vi "IB_RW_Project_RegGroup.vi"(7 "action":T3, 8 "error in (no error)":errorcluster, 9 "index in":string, 10 "RegGroup":T2, 11 "buildObject":T1) -> (0 "error out":errorcluster, 1 "index out":string, 2 "RegGroup":T2, 3 "buildObject out":T1)   [LabVIEW 2020]
doc: "Reads and writes the data to the object property bag."
uses:
  <resource>/Framework/Providers/API/ItemRef.ctl
  <vilib>/AppBuilder/IB_RW_Project/IB_RW_Project_PropBag_Action.ctl
  <vilib>/AppBuilder/IB_RW_Project/IB_RW_Project_RegGroup_Data.ctl
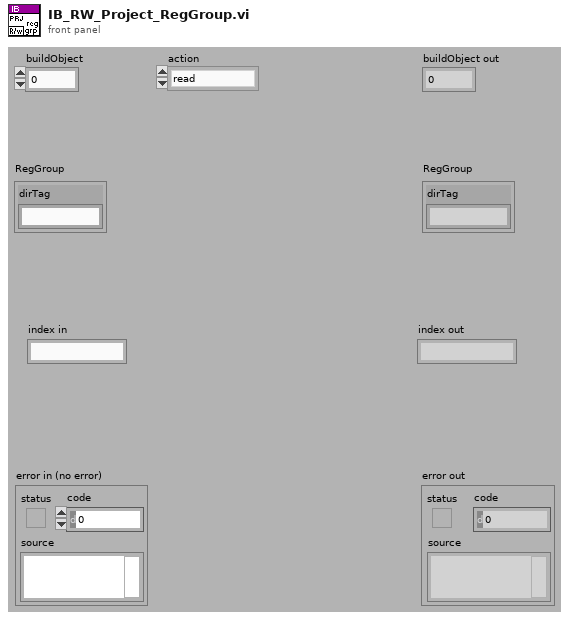
[diagram p1: front panel]
types:
  T1 = typedef "ItemRef.ctl" = u64
  T2 = typedef "IB_RW_Project_RegGroup_Data.ctl" = cluster{"dirTag":string}
  T3 = typedef "IB_RW_Project_PropBag_Action.ctl" = enum16{"read", "write", "clear", "readPrevious", "writePrevious", "clearPrevious"}
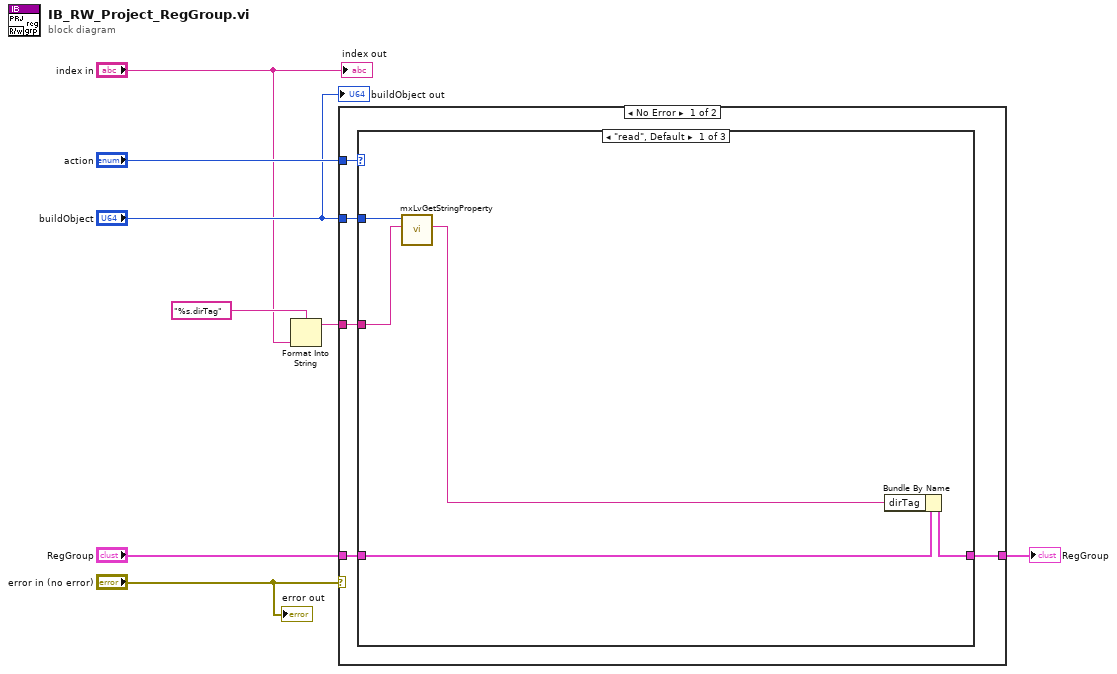
[diagram p0: block diagram]
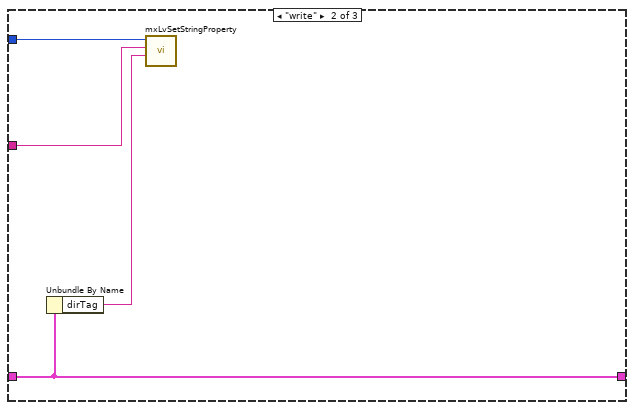
[diagram p2: hidden frame]
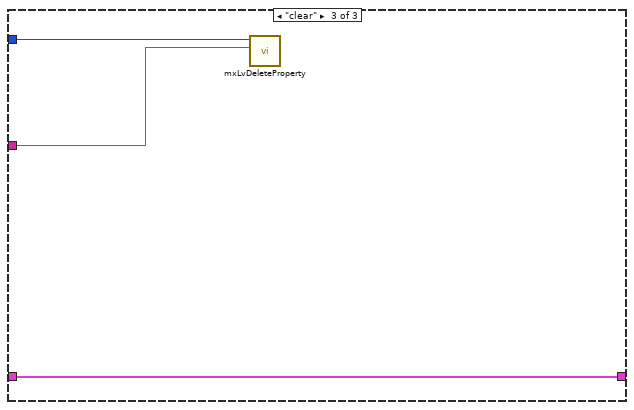
[diagram p3: hidden frame]
diagram:
  n1 = Format Into String(format string="%s.dirTag", "index in") -> (resulting string=w5:string)  [unwired: 2 in, 1 out]
  n2 = case shown="No Error" "error in (no error)" {
    tunnel: "action" -> [w13 _]
    tunnel: "RegGroup" -> [w12 w26]
    tunnel: w5 -> [w11 _]
    tunnel: [w10 w26] -> w4
    tunnel: "buildObject" -> [w9 _]
    frame No Error {
      n3 = case shown="\"read\", Default" w13 {
        tunnel: w9 -> [w16 w21 w24]
        tunnel: w12 -> [w18 w22 w25]
        tunnel: w11 -> [w15 w20 w23]
        tunnel: [w17 w22 w25] -> w10
        frame "read", Default {
          n4 = call <resource>:"mxLvGetStringProperty.vi"("Tag"=w15, "Item"=w16) -> ("Value"=w14:string)  [unwired: 1 in, 8 out]
          n5 = Bundle By Name(cluster=w18, "dirTag"=w14) -> (w17:T2)
        }
        frame "write" {
          n6 = Unbundle By Name(w22) -> ("dirTag"=w19:string)
          n7 = call <resource>:"mxLvSetStringProperty.vi"("Value (\"\")"=w19, "Tag"=w20, "Item"=w21) -> ()  [unwired: 2 in, 7 out]
        }
        frame "clear" {
          n8 = call <resource>:"mxLvDeleteProperty.vi"("Tag"=w23, "Item"=w24) -> ()  [unwired: 1 in, 9 out]
        }
      }
    }
    frame Error {
    }
  }
  "RegGroup" <- w4
  "error out" <- "error in (no error)"
  "buildObject out" <- "buildObject"
  "index out" <- "index in"
